vi "Track Limelight Target (X Axis).vi"() -> (2 "Joystick X":dbl)   [LabVIEW 2019]
uses:
  <vilib>/Rock Robotics/Network Tables/NT Read Number.vi
  <vilib>/addons/control/pid/pid.llb/PID (DBL).vi
  <vilib>/Rock Robotics/Network Tables/NT Write Number.vi
  Robot Global Data.vi
  <vilib>/addons/control/pid/NI_PID_pid.lvlib
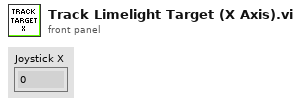
[diagram p1: front panel]
types:
  T1 = cluster{"proportional gain (Kc)":dbl, "integral time (Ti, min)":dbl, "derivative time (Td, min)":dbl}
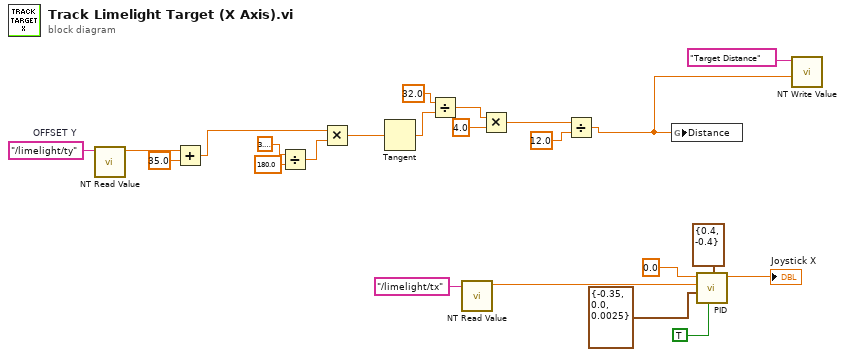
[diagram p0: block diagram]
diagram:
  w8 = "/limelight/ty"  # OFFSET Y
  n1 = call-poly <vilib>:"NT Read Value.vi"("Name"=w8) -> ("Numeric"=w10:dbl)  [unwired: 9 in, 1 out]
  n2 = Add(x=w10, y=35.0) -> (x+y=w12:dbl)
  n3 = Divide(x=3.141592653589793, y=180.0) -> (x/y=w3:dbl)
  n4 = Multiply(x=w12, y=w3) -> (x*y=w4:dbl)
  n5 = Tangent(1:w4) -> (0:w5:dbl)
  n6 = Divide(x=32.0, y=w5) -> (x/y=w13:dbl)
  n7 = call-poly <vilib>:"NT Read Value.vi"("Name"="/limelight/tx") -> ("Numeric"=w16:dbl)  [unwired: 9 in, 1 out]
  n8 = Multiply(x=w13, y=4.0) -> (x*y=w22:dbl)
  n9 = Divide(x=w22, y=12.0) -> (x/y=w1:dbl)
  n10 = global write "Robot Global Data.vi" "Distance"(w1) -> ()
  n11 = call-poly <vilib>:"PID.vi"("reinitialize? (F)"=TRUE, "output range"=cluster{"output high":dbl, "output low":dbl} {"output high"=0.4, "output low"=-0.4}, "PID gains"=T1 {"proportional gain (Kc)"=-0.35, "integral time (Ti, min)"=0.0, "derivative time (Td, min)"=0.0025}, "process variable"=w16, "setpoint"=0.0) -> ("output"=→"Joystick X":dbl)  [unwired: 5 in, 1 out]
  n12 = call-poly <vilib>:"NT Write Value.vi"("Numeric"=w1, "Name"="Target Distance") -> ()  [unwired: 9 in, 1 out]
